vi "MonitorUpdate.vi"(7 "LabVIEW Web Service Request":refnum<class "Web Request.lvclass">) -> ()   [LabVIEW 2014]
uses:
  <vilib>/wsapi/Web Request.lvclass
  <vilib>/picture/picture.llb/imagedata.ctl
  <vilib>/wsapi/NI_WebServices.lvlib
panel:
  # "Use the Web Service Request input terminal to call the VIs on the Web Services palette. Do not remove it from the connector pane unless you don't need access to the palette."
  # "Each additional control wired to the connector pane will be available as an input in the URL. To include an indicator in terminal-mode output (the default setting), it must also be wired to the connector pane."
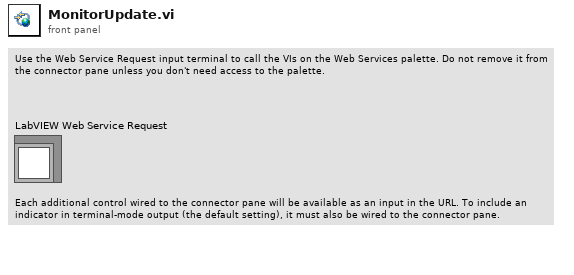
[diagram p1: front panel]
types:
  T1 = typedef "imagedata.ctl" = cluster{"image type":i32, "image depth":i32, "image":u8[], "mask":u8[], "colors":u32[], "Rectangle":cluster{"left":i16, "top":i16, "right":i16, "bottom":i16}}
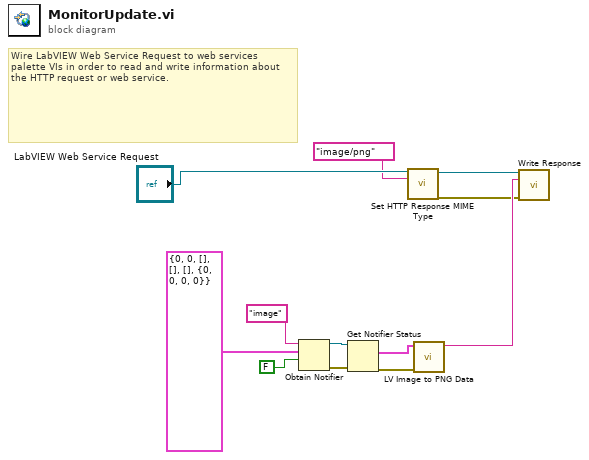
[diagram p0: block diagram]
diagram:
  # "Wire LabVIEW Web Service Request to web services palette VIs in order to read and write information about the HTTP request or web service."
  n1 = Obtain Notifier(name (unnamed)="image", notification data type=T1 {"image type"=0, "image depth"=0, "image"=[], "mask"=[], "colors"=[], "Rectangle"={"left"=0, "top"=0, "right"=0, "bottom"=0}} ("Image Data"), create if not found? (T)=FALSE) -> (notifier out=w9:refnum<notifier>, error out=w10:errorcluster)  [unwired: 1 in, 1 out]
  n2 = Get Notifier Status(notifier=w9, error in (no error)=w10) -> (current notification=w7:T1, error out=w6:errorcluster)  [unwired: 3 out]
  n3 = call <vilib>:"Set HTTP Response MIME Type.vi"("LabVIEW Web Service Request"="LabVIEW Web Service Request", "MIME type (text/html)"="image/png") -> ("LabVIEW Web Service Request out"=w3:refnum<class "Web Request.lvclass">, "error out"=w1:errorcluster)  [unwired: 12 in]
  n4 = call <vilib>:"LV Image to PNG Data.vi"("error in (no error)"=w6, "image data"=w7) -> ("png data"=w2:string)  [unwired: 8 in, 1 out]
  n5 = call <vilib>:"Write Response.vi"("LabVIEW Web Service Request"=w3, "response string"=w2, "error in (no error)"=w1) -> ()  [unwired: 11 in, 2 out]
